vi "Test DRAM Throughput.vi"(7 "fifo depth":u8(ring)=16 items=["4"=2, "8"=3, "16"=4, "32"=5, "64"=6, "128"=7, "256"=8, "512"=9, "1024"=10, "2048"=11, "4096"=12, "8192"=13, "16384"=14, "32768"=15, "65536"=16, "131072"=17, "262144"=18, "524288"=19, "1048576"=20, "2097152"=21, "4194304"=22, "8388608"=23, "16777216"=24, "33554432"=25, "67108864"=26, "134217728"=27, "268435456"=28, "536870912"=29, "1073741824"=30, "2147483648"=31, "4294967296"=32], 10 "arbiter configuration":T3={"write grant time (clocks)"=100, "read grant time (clocks)"=100}, 11 "Points to Generate":u32=100 format="%.0p") -> (2 "Pass?":bool, 3 "Write Throughput (Bytes/sec)":u32 format="%.2p")   [LabVIEW 2011]
uses:
  <instrlib>/FlexRIO/Libraries/Memory/FPGA/Interface/Timeslot Arbiter Configuration.ctl
  <instrlib>/RF-RIO/FIFO/FIFO/FPGA/Public/FIFO State.ctl
  <vilib>/Platform/TimedLoop/XDataNode/timing_clust.ctl
  <vilib>/Platform/TimedLoop/XDataNode/nitl_modes.ctl
  <vilib>/Platform/TimedLoop/XDataNode/wakeup.ctl
  <vilib>/Platform/TimedLoop/XDataNode/XDataNode.xnode
  <instrlib>/RF-RIO/FIFO/FIFO/FPGA/FIFO.lvlib
  <vilib>/Platform/TimedLoop/XDataNode/XDNodeRunTimeDep.lvlib
  <instrlib>/FlexRIO/Libraries/Memory/FPGA/Memory.lvlib
panel:
  out "Generation Done Ticks":i32
  out "DRAM Retrieval in Ticks":u32
  out "count 2":u32
  out "state":T1
  out "count":u32
  out "bank1.data":T2
  out "bank0.data":T2
  out "Last Address Failed":u32
  out "Points Read from FIFO":u32
  out "Read Throughput (Bytes/sec)":u32 format="%.2p"
  out "Gen. Points Done":u32 format="%.0p"
  out "Generation Done?":bool
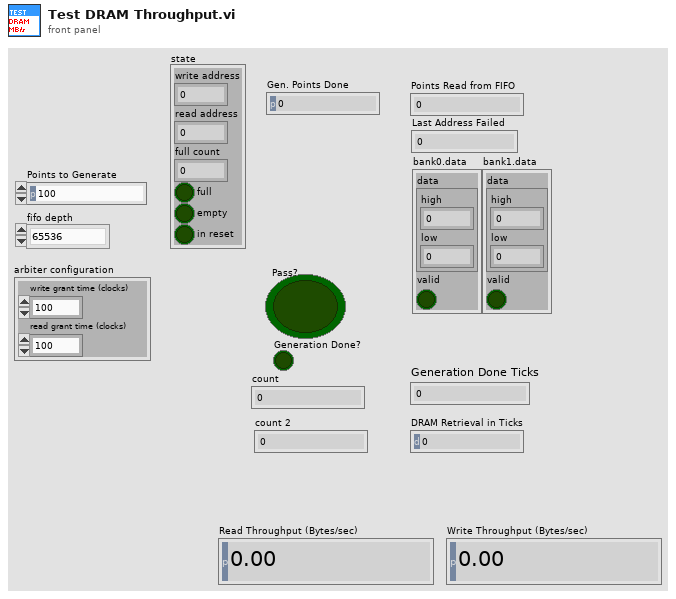
[diagram p1: front panel]
types:
  T1 = typedef "FIFO.lvlib/FIFO State.ctl" = cluster{"write address":u32, "read address":u32, "full count":u32, "full":bool, "empty":bool, "in reset":bool}
  T2 = cluster{"data":cluster{"high":u64, "low":u64}, "valid":bool}
  T3 = typedef "Memory.lvlib/Timeslot Arbiter Configuration.ctl" = cluster{"write grant time (clocks)":u16, "read grant time (clocks)":u16}
  T4 = typedef "XDNodeRunTimeDep.lvlib/timing_clust.ctl" = cluster{"Expected End [f-1]":u64, "Actual End [f-1]":u64, "Finished Late? [f-1]":bool, "Expected End [i-1]":u64, "Actual End [i-1]":u64, "Finished Late? [i-1]":bool, "Expected Start [i]":u64, "Actual Start [i]":u64, "Expected Start [f]":u64, "Actual Start [f]":u64, "Source Name":string, "Structure Name":string, "Period":i64, "Deadline":i64, "Offset":i64, "Start":i64, "Priority":i32, "Timeout":i32, "Mode":T5, "Wakeup Reason":T6, "Error":errorcluster, "Source Type":string, "Secondary Source Type":string, "Global End Time":u64, "Global Start Time":u64, "Frame Duration":u64, "Iteration Duration":u64, "Assigned CPU":i32, "I/O Scan Engine Mode":u32}
  T5 = typedef "XDNodeRunTimeDep.lvlib/nitl_modes.ctl" = enum32{"No Change", "Process missed periods, maintain original phase", "Discard missed periods, maintain original phase", "Process missed periods, ignore original phase", "Discard missed periods, ignore original phase"}
  T6 = typedef "XDNodeRunTimeDep.lvlib/wakeup.ctl" = enum32{"Normal", "Aborted", "Asynchronous wakeup", "Timing source error", "Timed loop error", "Timeout"}
  T7 = cluster{"fifo1 memory":refnum<k21>, "fifo2 memory":refnum<k21>}
  T8 = typedef "Data Type (256).ctl" = cluster{"Bank0. High":u64, "Bank0. Low":u64, "Bank1. High":u64, "Bank1. Low":u64}
  T9 = typedef "FIFO.lvlib/niRFRIO Memory 1.0.0 FPGA.lvlib/Retrieve Data (128-Bit).ctl" = cluster{"data":T10, "valid":bool}
  T10 = typedef "FIFO.lvlib/niRFRIO Memory 1.0.0 FPGA.lvlib/U128.ctl" = cluster{"high":u64, "low":u64}
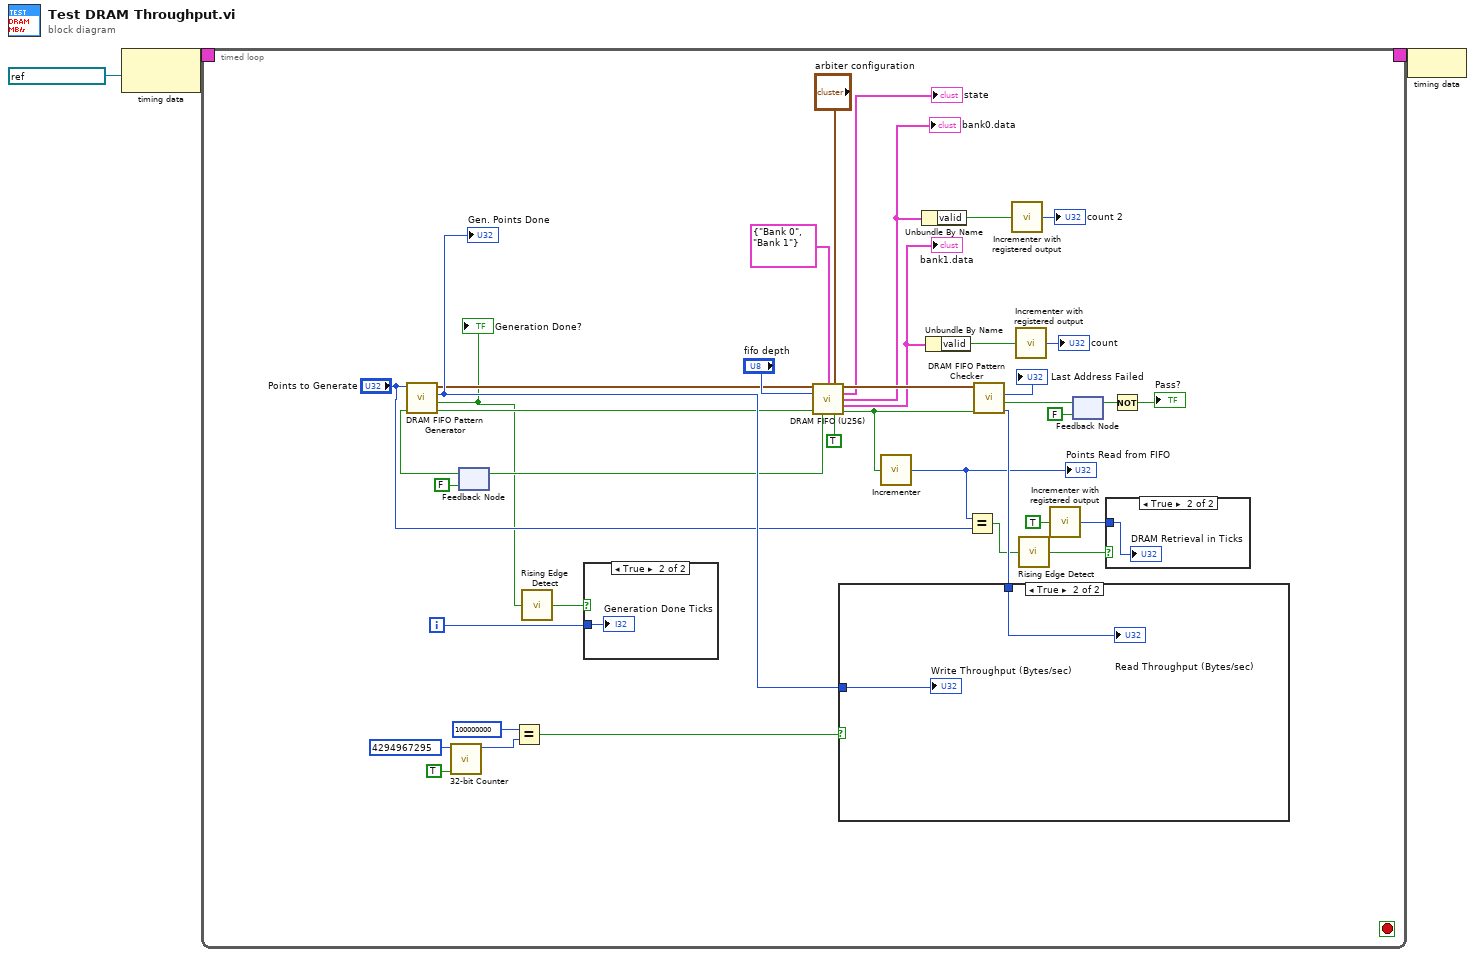
[diagram p0: block diagram]
diagram:
  n1 = node-c288(refnum<k21> "100 MHz Clock" ("Source Name")) -> (w3:T4)
  n2 = timed-loop {
    timing: w3 -> [_]
    timing-out: [_] -> w2
    i -> [w6]
    stop <- _ stop-if-true
    n3 = call <userlib>:"32-bit Counter.vi"("INC?"=TRUE, "rollover"=u32 4294967295) -> ("count"=w31:u32)  [unwired: 9 in]
    n4 = feedback #1(FALSE ("Ready for Input")) -> (w41:bool)
    n5 = call <userlib>:"DRAM FIFO Pattern Generator.vi"("Generate Point"=w41, "Points to Generate"="Points to Generate") -> ("Output Valid"=w7:bool, "Generation Done?"=w5:bool, "Points Done"=w27:u32, "Output Data"=w18:T8)  [unwired: 6 in]
    "Generation Done?" <- w5
    "Gen. Points Done" <- w27
    n6 = Equal?(x=u32 100000000, y=w31) -> (x = y?=w32:bool)
    n7 = call <userlib>:"Rising Edge Detect.vi"("signal"=w5) -> ("edge detected"=w4:bool)  [unwired: 14 in]
    n8 = case shown="True" w4 {
      tunnel: w6 -> [_ w43]
      frame False {
      }
      frame True {
        "Generation Done Ticks" <- w43
      }
    }
    n9 = call <userlib>:"DRAM FIFO (U256).vi"("Input Data"=w18, "Memory"=T7 {"fifo1 memory"="Bank 0", "fifo2 memory"="Bank 1"}, "arbiter configuration"="arbiter configuration", "fifo depth"="fifo depth", "input valid"=w7, "ready for output"=TRUE) -> ("Output Data"=w35:T8, "state"=→"state":T1, "bank0.data"=w16:T9, "Bank1.data"=w14:T9, "Ready for Input"=w25:bool, "Output Valid"=w23:bool)  [unwired: 4 in]
    "bank0.data" <- w16
    "bank1.data" <- w14
    n10 = feedback-in #1(w25) -> ()
    n11 = call <userlib>:"Incrementer.vi"("INC?"=w23) -> ("count"=w13:u32)  [unwired: 4 in]
    "Points Read from FIFO" <- w13
    n12 = Unbundle By Name(w16) -> ("valid"=w17:bool)
    n13 = Unbundle By Name(w14) -> ("valid"=w15:bool)
    n14 = Equal?(x=w13, y="Points to Generate") -> (x = y?=w9:bool)
    n15 = call <userlib>:"DRAM FIFO Pattern Checker.vi"("Input Valid"=w23, "Input Data"=w35) -> ("Points Done"=w26:u32, "Pattern Match Ever Fail?"=w40:bool, "Last Address Failed"=→"Last Address Failed":u32)  [unwired: 3 in, 4 out]
    n16 = case shown="True" w32 {
      tunnel: w27 -> [_ w46]
      tunnel: w26 -> [_ w45]
      frame False {
      }
      frame True {
        "Write Throughput (Bytes/sec)" <- w46
        "Read Throughput (Bytes/sec)" <- w45
      }
    }
    n17 = call <userlib>:"Incrementer with registered output.vi"("INC?"=w17) -> ("count"=→"count 2":u32)  [unwired: 4 in]
    n18 = call <userlib>:"Incrementer with registered output.vi"("INC?"=w15) -> ("count"=→"count":u32)  [unwired: 4 in]
    n19 = call <userlib>:"Rising Edge Detect.vi"("signal"=w9) -> ("edge detected"=w8:bool)  [unwired: 14 in]
    n20 = call <userlib>:"Incrementer with registered output.vi"("INC?"=TRUE) -> ("count"=w11:u32)  [unwired: 4 in]
    n21 = feedback #2(FALSE ("Pattern Match Ever Fail?")) -> (w34:bool)
    n22 = feedback-in #2(w40) -> ()
    n23 = case shown="True" w8 {
      tunnel: w11 -> [_ w44]
      frame False {
      }
      frame True {
        "DRAM Retrieval in Ticks" <- w44
      }
    }
    n24 = Not(x=w34) -> (.not. x?=→"Pass?":bool)
  }
  n25 = node-c288(w2) -> ()
